vi "LV2017CP.vi"() -> ()   [LabVIEW 2016]
doc: "This example performs a serial port write and a serial port read. The parameters set for the serial port must match the parameters of the connected instrument or device. The VISA Configure Serial Port VI sets the configuration parameters. The front panel displays the controls used to configure the basic parameters, such as baud rate, data bits, and parity. The VI passes the VISA resource name to other VIs that perform operations on that VISA resource. The VISA Write function sends a command to the serial device and the VISA Read function returns data based on the command. The VISA Close function then closes the reference to the serial device. It is important to close the reference; otherwise, further communication through that port might not be possible."
uses:
  <vilib>/Instr/_visa.llb/VISA Configure Serial Port (Instr).vi
  Serial - Settings.ctl
panel:
  in  "Tyre Diameter(m) 2":sgl=0.5
  in  "Name your log file:":string="09_12_2019"
  in  "Error Cancellation (Def:On)":bool
  out "Answer to Write Command 2":string
  out "Speed Reference":sgl(graph)=57.306286
  out "Speed Ref in 21202":string
  out "Floating Point 5":sgl
  out "Speed Ref in 21201":string
  in  "write buffer 5":string="\u0002\u0003RÑ\u0000\u0002„¹"
  out "Floating Point 4":sgl
  out "Speed Ref in 21201":string
  in  "write buffer 4":string="\u0002\u0003RÐ\u0000\u0002Õy"
  in  "write buffer 3":string="\u0002\u0003I<\u0000\u0002\u0012h"
  out "read buffer 6":string
  out "read buffer 5":string
  out "read buffer 4":string
  out "read buffer 3":string
  out "read buffer 2":string
  out "read buffer":string
  in  "write buffer 2":string="\u0002\u0003RÏ\u0000\u0002ä¿"
  in  "write buffer":string="\u0002\u0010RÏ\u0000\u0002\u0004\u0000\u0000@ d "
  out "Answer to Write Command":string
  out "Floating Point 3":sgl=5.00679
  out "Speed Ref in 21200":string
  out "Floating Point 2":sgl=0.14305113
  out "Speed Ref in Monitor":string
  out "I_d":sgl(graph)=0.08283757
  out "I_q":sgl(graph)=-0.08283757
  out "Power(kW)":sgl(graph)=8.934696e-07
  out "Current(I)":sgl(graph)
  in  "file path (dialog if empty)":path=path "C:/Users/arda/Desktop/Thesis/random.txt"
  in  "Tyre Diameter(m)":sgl=0.5
  out "Measured RPM":sgl(graph)
  in  "Enum":T1(ring)=enum."Default"
  in  "Continuous Connection(Def:ON)":bool=TRUE
  out "Estimated Torque":sgl(graph)=-0.29821524
  in  "Finish session(Def:Off/False)":bool
  in  "Connectivity Check (Def:Off)":bool
  in  "timeout (10sec)":u32=10000
  out "connection check":u8[](array[numeric])=[0, 0, 0, 2]
  in  "Enable Termination\nChar (T)":bool
  in  "connection_verification":string="\u0002\u0003Fm\u0000\u0002@­"
  out "Serial Settings:Wire Mode":i8(ring)=-128 items=["Unknown"=-1, "RS485/Wire4"=0, "RS485/Wire2-EchoDTR"=1, "RS485/Wire2-CtrlDTR"=2, "RS485/Wire2-Auto"=3, "RS232/DTE"=-128, "RS232/DCE"=-127, "RS232/Auto"=-126]
  out "message":string="No Error"
  in  "Serial Settings":T2={"baud rate"=19200, "data bits"=8, "parity"=enum."Even", "stop bits"=10, "flow control"=0} {"flow control" items=["None"=0, "XON/XOFF"=1, "RTS/CTS"=2, "DTR/DSR"=4]; "stop bits" items=["1.0"=10, "1.5"=15, "2.0"=20]; "data bits" min=5 max=8 step=1; "baud rate" items=["75"=75, "110"=110, "134"=134, "150"=150, "300"=300, "600"=600, "1200"=1200, "1800"=1800, "2400"=2400, "4800"=4800, "9600"=7200, "19600"=9600, "14400"=14400, "19200"=19200, "28800"=28800, "38400"=38400, "56000"=56000, "57600"=57600, "115200"=115200, "128000"=128000, "230400"=230400]}
  in  "VISA resource name":refnum<visa-resource-name>="COM8"
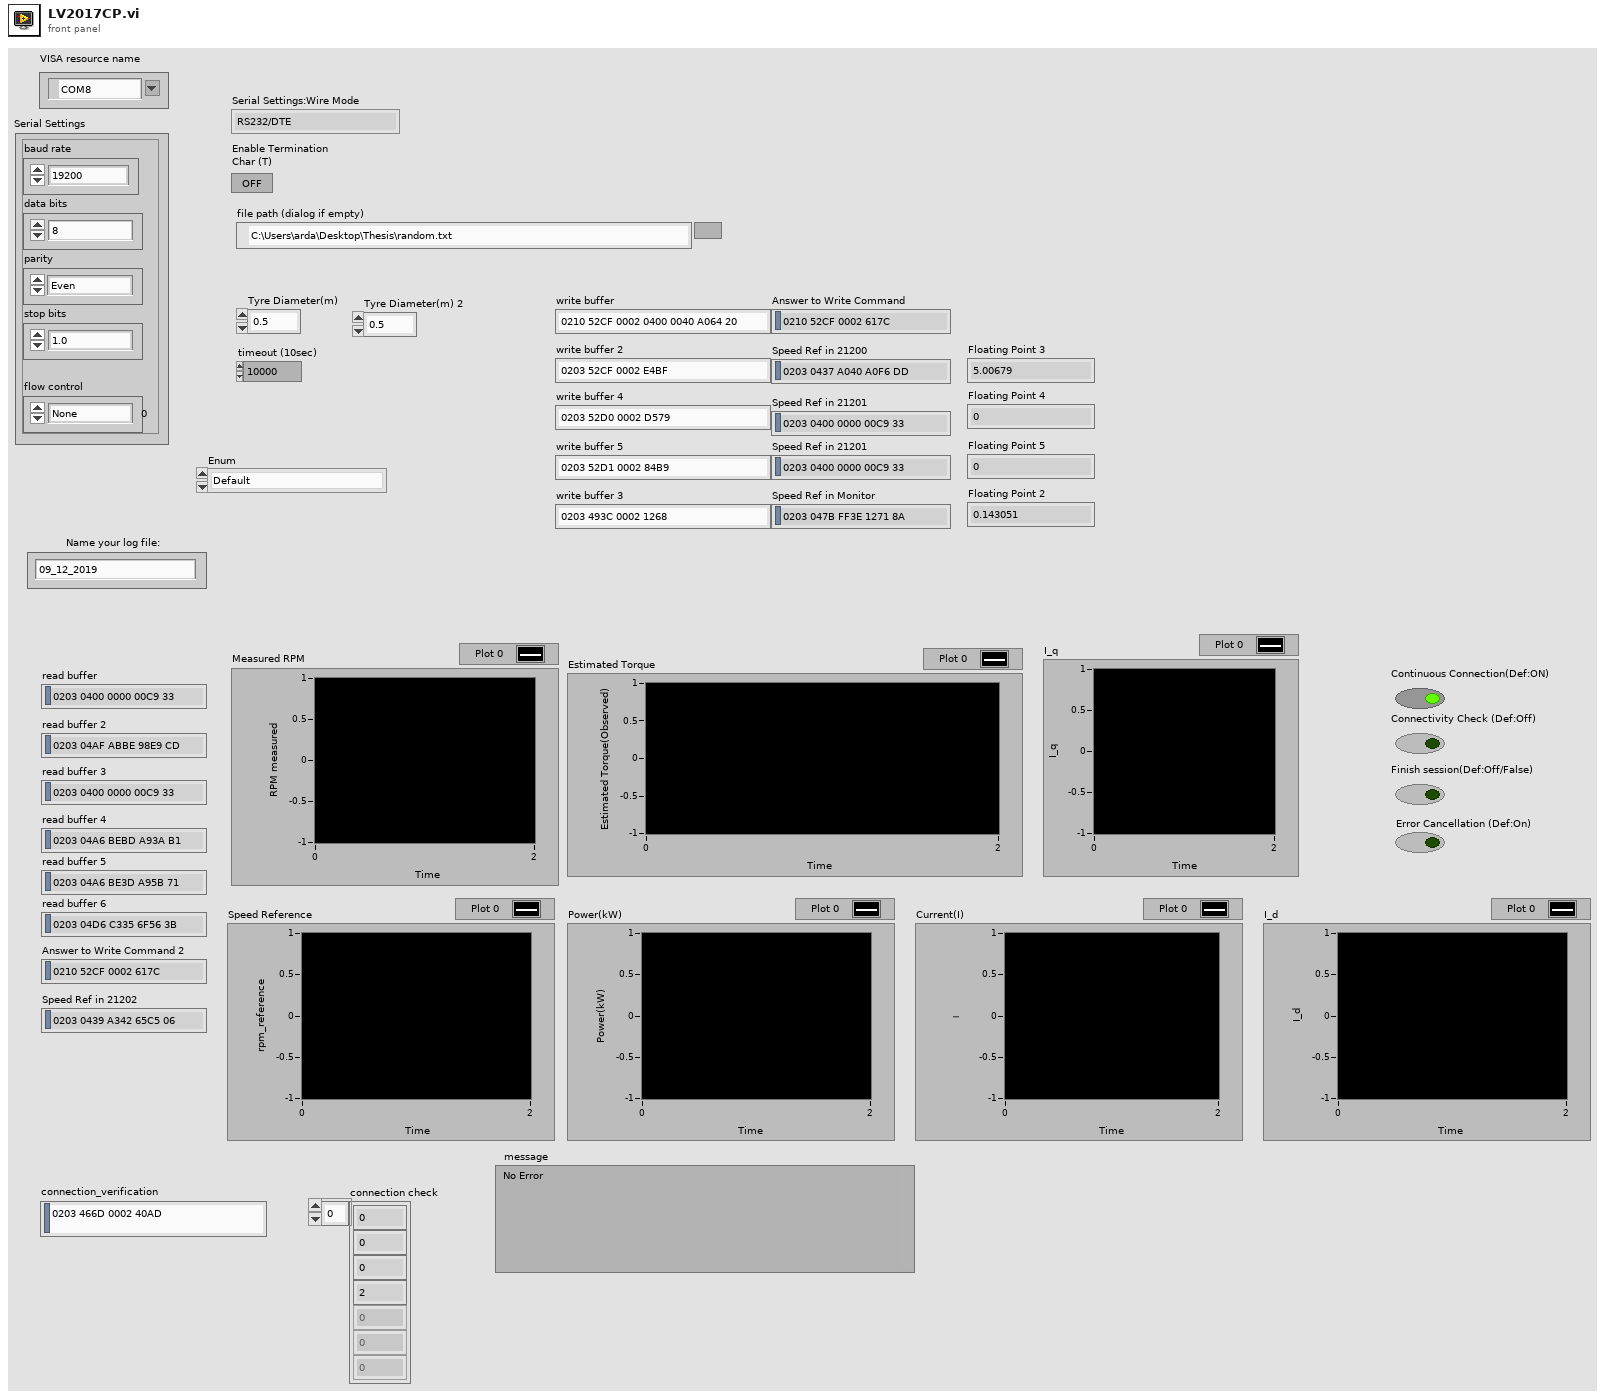
[diagram p1: front panel]
types:
  T1 = enum16{"Single Signal Trials", "Default", "Alarm Reset", "Write Save Command", "Drive Reset"}
  T2 = typedef "Serial - Settings.ctl" = cluster{"baud rate":u32, "data bits":u16, "parity":enum16{"None", "Odd", "Even", "Mark", "Space"}, "stop bits":u16, "flow control":u16}
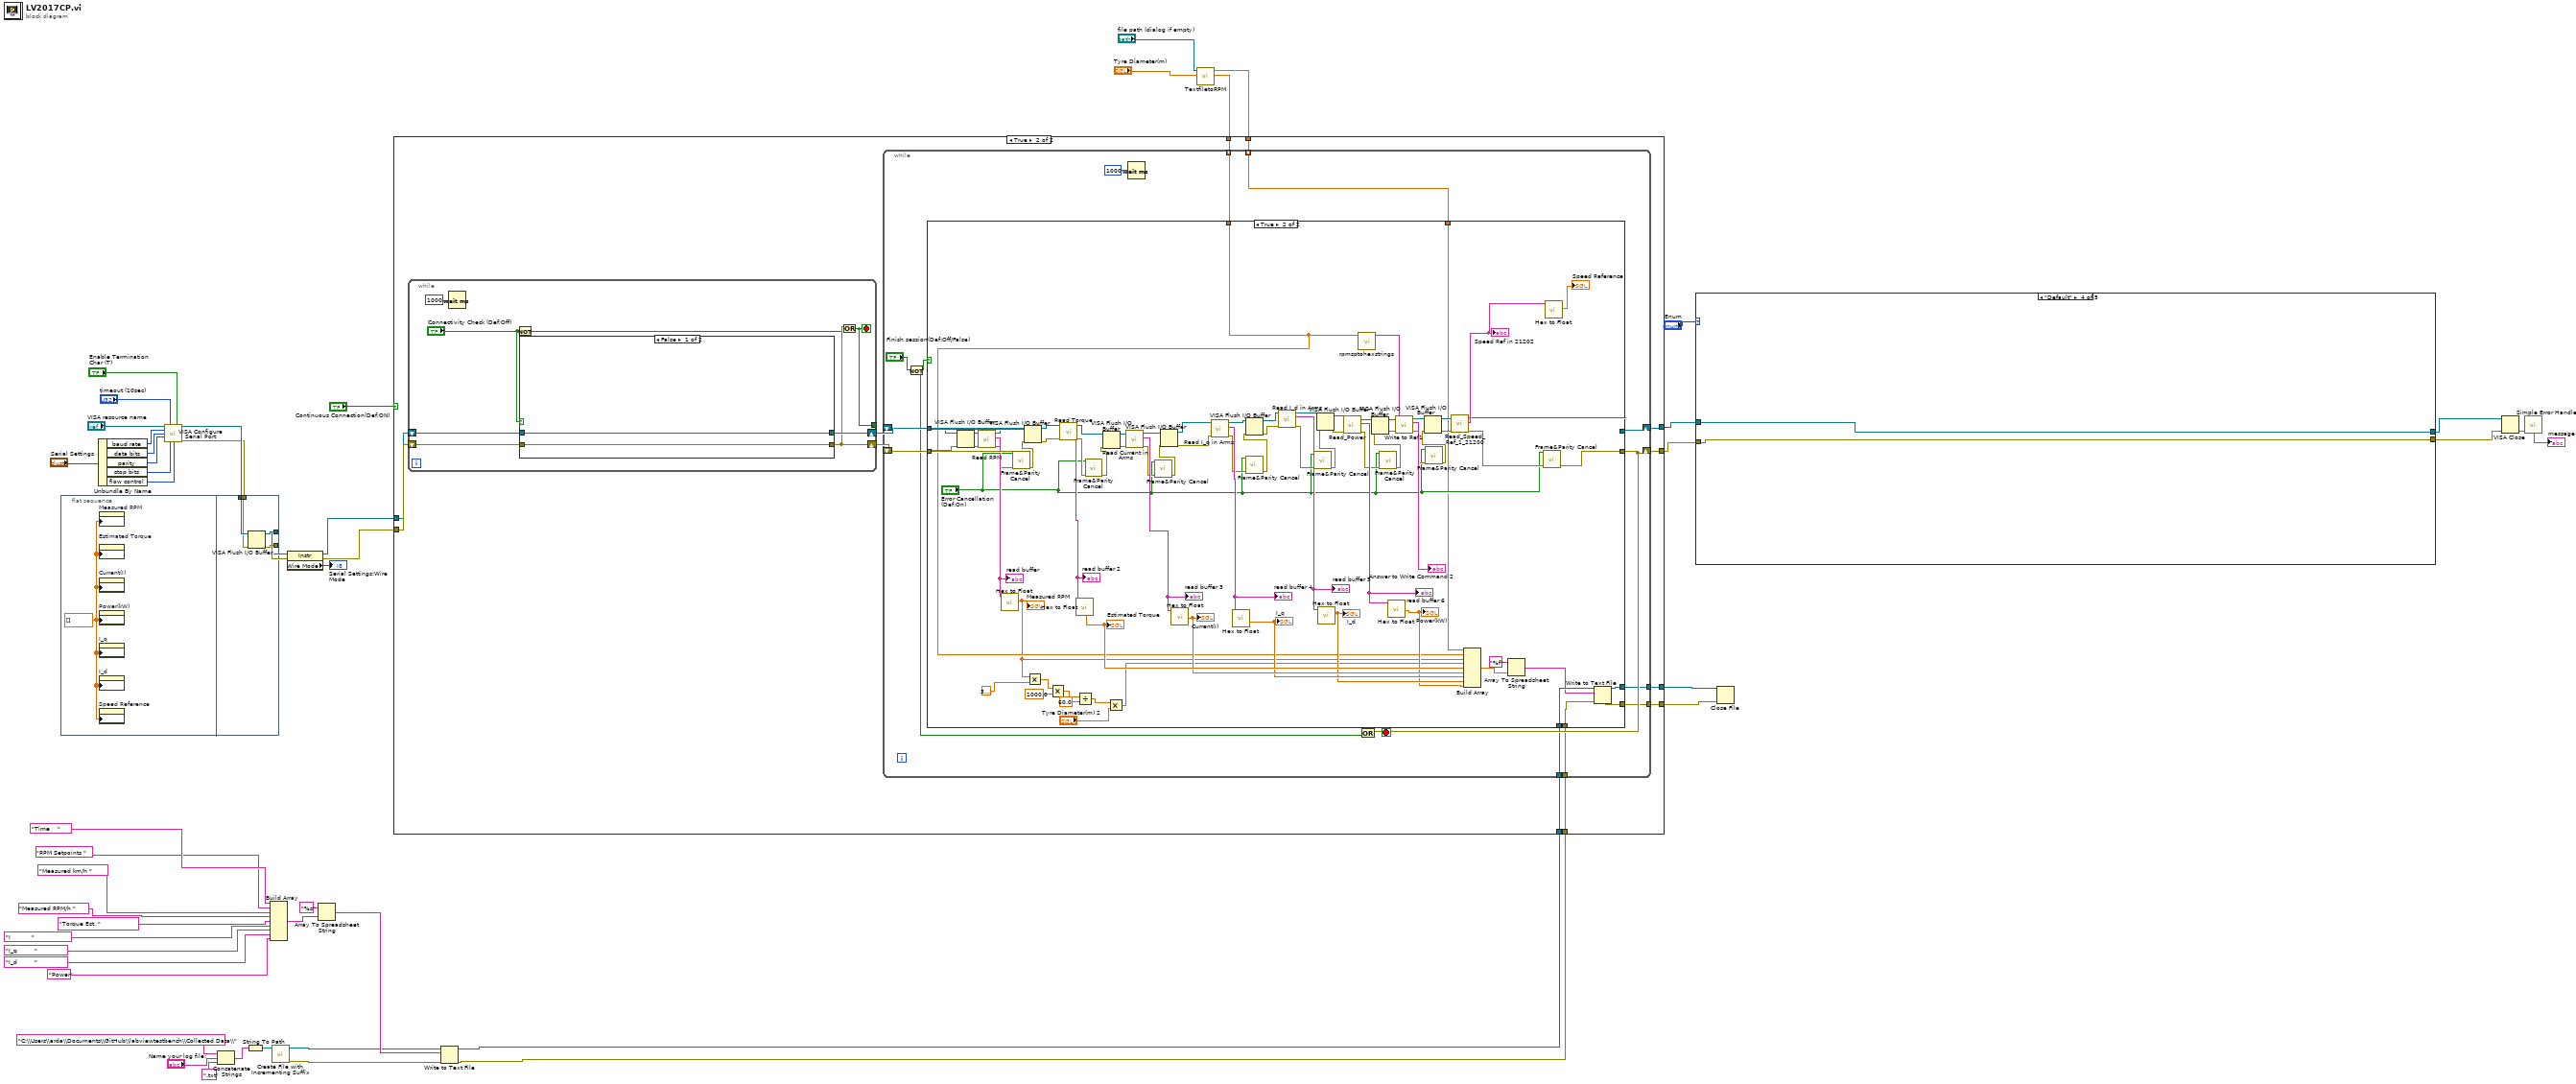
[diagram p0: block diagram]
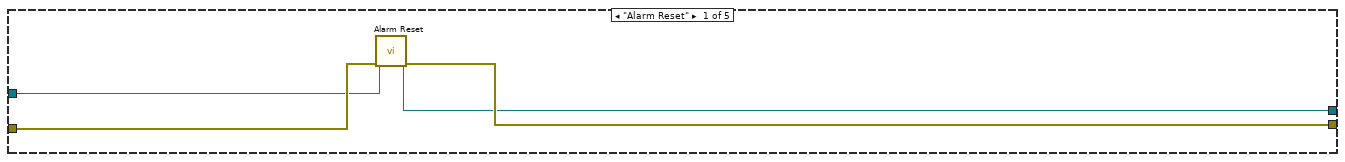
[diagram p2: hidden frame]
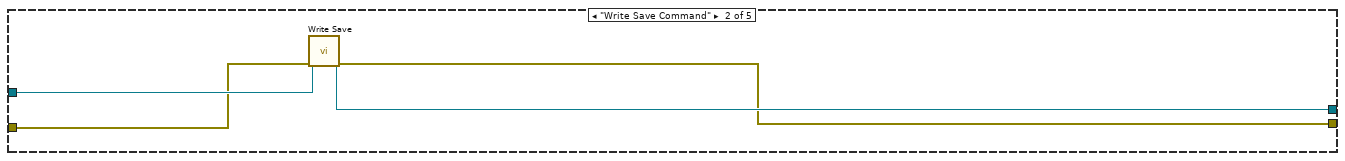
[diagram p3: hidden frame]
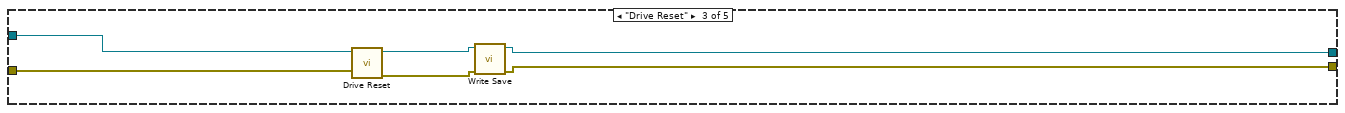
[diagram p4: hidden frame]
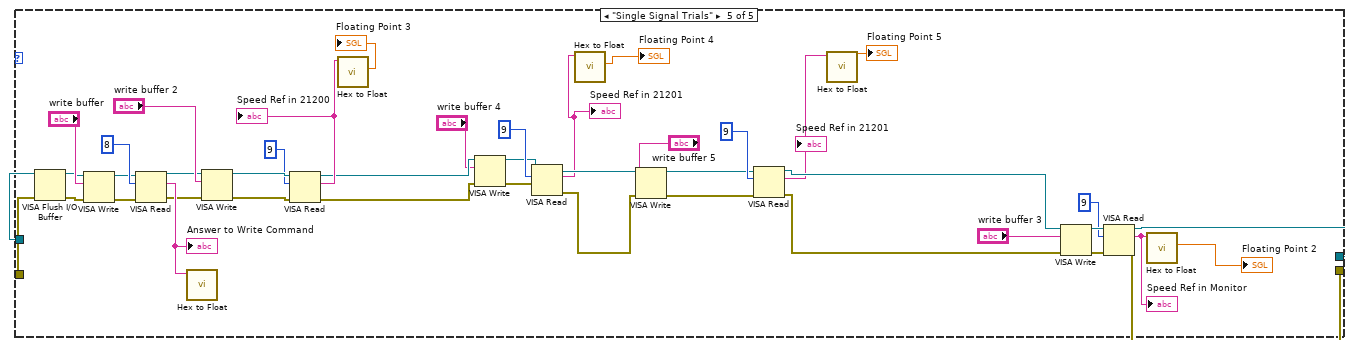
[diagram p5: hidden frame]
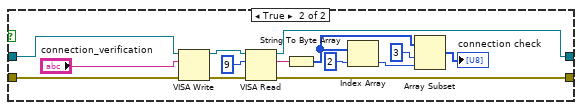
[diagram p7: hidden frame]
diagram:
  n1 = flat-sequence {
    tunnel: [w56] -> w42
    tunnel: [w55] -> w41
    tunnel: w40 -> [w54]
    tunnel: w39 -> [w53]
    frame #0 {
      w52 = sgl[] [] ("History Data")
      n2 = property on="Measured RPM" class="WFChart (strict)"("History Data"=w52) -> ()  [unwired: 2 in, 2 out]
      n3 = property on="Estimated Torque" class="WFChart (strict)"("History Data"=w52) -> ()  [unwired: 2 in, 2 out]
      n4 = property on="Current(I)" class="WFChart (strict)"("History Data"=w52) -> ()  [unwired: 2 in, 2 out]
      n5 = property on="Power(kW)" class="WFChart (strict)"("History Data"=w52) -> ()  [unwired: 2 in, 2 out]
      n6 = property on="I_q" class="WFChart (strict)"("History Data"=w52) -> ()  [unwired: 2 in, 2 out]
      n7 = property on="I_d" class="WFChart (strict)"("History Data"=w52) -> ()  [unwired: 2 in, 2 out]
      n8 = property on="Speed Reference" class="WFChart (strict)"("History Data"=w52) -> ()  [unwired: 2 in, 2 out]
    }
    frame #1 {
      n9 = VISA Flush I/O Buffer(VISA resource name=w54, error in (no error)=w53) -> (VISA resource name out=w55:refnum<visa-resource-name>, error out=w56:errorcluster)  [unwired: 1 in]
    }
  }
  n10 = Unbundle By Name("Serial Settings") -> ("baud rate"=w45:u32, "data bits"=w49:u16, "parity"=w48:enum16{"None", "Odd", "Even", "Mark", "Space"}, "stop bits"=w47:u16, "flow control"=w46:u16)
  n11 = call-poly "VISA Configure Serial Port"("VISA resource name"="VISA resource name", "timeout (10sec)"="timeout (10sec)", "Enable Termination\nChar (T)"="Enable Termination\nChar (T)", "baud rate (9600)"=w45, "data bits (8)"=w49, "parity (0:none)"=w48, "stop bits (10: 1 bit)"=w47, "flow control (0:none)"=w46) -> ("VISA resource name out"=w40:refnum<visa-resource-name>, "error out"=w39:errorcluster)  [unwired: 1 in, 5 out]
  n12 = Concatenate Strings("C:\\Users\\arda\\Documents\\GitHub\\labviewtestbench\\Collected Data\\" ("string"), "Name your log file:", ".txt") -> (w19:string)
  n13 = String To Path(string=w19) -> (path=w15:path)
  n14 = Build Array("Time    " ("element"), "RPM Setpoints ", "Measured km/h ", "Measured RPM/h ", "Torque Est. ", "I           " ("element"), "I_q         " ("element"), "I_d         " ("element"), "Power" ("element")) -> (w22:string[])
  n15 = call <vilib>:"Create File with Incrementing Suffix.vi"("file path"=w15) -> ("error out"=w13:errorcluster, "refnum out"=w14:refnum<file>)  [unwired: 8 in, 1 out]
  n16 = property class="Instr"(reference=w41, error in=w42) -> (reference out=w36:refnum<visa-resource-name>, error out=w37:errorcluster, "Wire Mode"=→"Serial Settings:Wire Mode":i16)
  n17 = Array To Spreadsheet String(array=w22, 3:"%s" ("format string")) -> (spreadsheet string=w20:string)  [unwired: 1 in]
  n18 = Write to Text File(file (use dialog)=w14, text=w20, error in=w13) -> (refnum out=w6:refnum<file>, error out=w7:errorcluster)  [unwired: 1 in, 1 out]
  n19 = call "TextfiletoRPM.vi"("Tyre Diameter(m)"="Tyre Diameter(m)", "file path (dialog if empty)"="file path (dialog if empty)") -> ("Array"=w28:dbl[], "time_sp"=w5:sgl[])  [unwired: 8 in]
  n20 = case shown="True" "Continuous Connection(Def:ON)" {
    tunnel: w37 -> [w59 w72]
    tunnel: w36 -> [w60 w71]
    tunnel: [w60 w68] -> w33
    tunnel: w28 -> [_ w67]
    tunnel: [w59 w66] -> w25
    tunnel: w6 -> [w57 w65]
    tunnel: w7 -> [w58 w64]
    tunnel: [w57 w63] -> w24
    tunnel: [w58 w62] -> w23
    tunnel: w5 -> [_ w61]
    frame False {
    }
    frame True {
      n21 = while {
        shift-right: [w80] -> w70
        shift-left: w71 -> [w79]
        shift-right: [w77] -> w69
        shift-left: w72 -> [w78]
        tunnel: [w73] -> _
        stop <- w73 stop-if-true
        n22 = Wait (ms)(milliseconds to wait=u32 1000) -> ()  [unwired: 1 out]
        n23 = Not(x="Connectivity Check (Def:Off)") -> (.not. x?=w74:bool)
        n24 = case shown="False" "Connectivity Check (Def:Off)" {
          tunnel: [w82 w96] -> w80
          tunnel: w79 -> [w82 w95]
          tunnel: w78 -> [w81 w94]
          tunnel: [w81 w93] -> w77
          frame False {
          }
          frame True {
            n25 = VISA Write(VISA resource name=w95, write buffer="connection_verification", error in (no error)=w94) -> (VISA resource name out=w92:refnum<visa-resource-name>, error out=w90:errorcluster)  [unwired: 1 out]
            n26 = VISA Read(VISA resource name=w92, byte count=u32 9, error in (no error)=w90) -> (VISA resource name out=w96:refnum<visa-resource-name>, read buffer=w84:string, error out=w93:errorcluster)  [unwired: 1 out]
            n27 = String To Byte Array(string=w84) -> (unsigned byte array=w88:u8[])
            n28 = Index Array(array=w88, index=2) -> (element=w85:u8)
            n29 = Array Subset(array=w88, index=3 ("length"), length=w85) -> (→"connection check":u8[])
          }
        }
        n30 = Or(x=w77, y=w74) -> (x .or. y?=w73:bool)
      }
      n31 = while {
        shift-right: [w108] -> w68
        shift-left: w70 -> [w110]
        shift-right: [w106] -> w66
        shift-left: w69 -> [w109]
        tunnel: w67 -> [w104] mode=indexing
        tunnel: w65 -> [w101]
        tunnel: w64 -> [w100]
        tunnel: [w99] -> w63
        tunnel: [w98] -> w62
        tunnel: w61 -> [w97] mode=indexing
        stop <- w105 stop-if-true
        n32 = Not(x="Finish session(Def:Off/False)") -> (.not. x?=w103:bool)
        n33 = case shown="True" w103 {
          tunnel: w110 -> [w114 w183]
          tunnel: w109 -> [w113 w181]
          tunnel: [w114 w177] -> w108
          tunnel: [w113 w184] -> w106
          tunnel: w104 -> [_ w117]
          tunnel: w101 -> [w112 w130]
          tunnel: w100 -> [w111 w129]
          tunnel: [w112 w128] -> w99
          tunnel: [w111 w127] -> w98
          tunnel: w97 -> [_ w118]
          frame False {
          }
          frame True {
            n34 = VISA Flush I/O Buffer(VISA resource name=w183, error in (no error)=w181) -> (VISA resource name out=w182:refnum<visa-resource-name>, error out=w174:errorcluster)  [unwired: 1 in]
            n35 = call "Read RPM.vi"("error in (no error)"=w174, "VISA resource name"=w182) -> ("error out"=w152:errorcluster, "read buffer"=w189:string, "VISA resource name out"=w173:refnum<visa-resource-name>)  [unwired: 7 in]
            "read buffer" <- w189
            n36 = call "Hex to Float.vi"("read buffer in"=w189) -> ("Floating Point"=w116:sgl)  [unwired: 9 in, 1 out]
            "Measured RPM" <- w116
            n37 = call "Frame&Parity Cancel.vi"("error in (no error)"=w152, "Error Cancellation (Def:On)"="Error Cancellation (Def:On)") -> ("error out"=w151:errorcluster)  [unwired: 9 in]
            n38 = VISA Flush I/O Buffer(VISA resource name=w173, error in (no error)=w151) -> (VISA resource name out=w172:refnum<visa-resource-name>, error out=w171:errorcluster)  [unwired: 1 in]
            n39 = Multiply(x=w116, y=3.141592653589793) -> (x*y=w124:dbl)
            n40 = Multiply(x=w124, y=1000.0) -> (x*y=w122:dbl)
            n41 = call "Read Torque.vi"("error in (no error)"=w171, "VISA Refnum in"=w172) -> ("error out"=w150:errorcluster, "read buffer"=w190:string, "VISA Refnum out"=w170:refnum<visa-resource-name>)  [unwired: 7 in]
            "read buffer 2" <- w190
            n42 = call "Hex to Float.vi"("read buffer in"=w190) -> ("Floating Point"=w137:sgl)  [unwired: 9 in, 1 out]
            "Estimated Torque" <- w137
            n43 = Divide(x=w122, y=60.0) -> (x/y=w120:dbl)
            n44 = call "Frame&Parity Cancel.vi"("error in (no error)"=w150, "Error Cancellation (Def:On)"="Error Cancellation (Def:On)") -> ("error out"=w149:errorcluster)  [unwired: 9 in]
            n45 = VISA Flush I/O Buffer(VISA resource name=w170, error in (no error)=w149) -> (VISA resource name out=w168:refnum<visa-resource-name>, error out=w169:errorcluster)  [unwired: 1 in]
            n46 = Multiply(x=w120, y="Tyre Diameter(m) 2") -> (x*y=w115:dbl)
            n47 = call "Read Current in Arms.vi"("error in (no error)"=w169, "VISA Refnum in"=w168) -> ("error out"=w148:errorcluster, "read buffer"=w187:string, "VISA Refnum out"=w167:refnum<visa-resource-name>)  [unwired: 7 in]
            "read buffer 3" <- w187
            n48 = call "Frame&Parity Cancel.vi"("error in (no error)"=w148, "Error Cancellation (Def:On)"="Error Cancellation (Def:On)") -> ("error out"=w147:errorcluster)  [unwired: 9 in]
            n49 = VISA Flush I/O Buffer(VISA resource name=w167, error in (no error)=w147) -> (VISA resource name out=w166:refnum<visa-resource-name>, error out=w165:errorcluster)  [unwired: 1 in]
            n50 = call "Hex to Float.vi"("read buffer in"=w187) -> ("Floating Point"=w136:sgl)  [unwired: 9 in, 1 out]
            "Current(I)" <- w136
            n51 = call "Read I_q in Arms.vi"("error in (no error)"=w165, "VISA Refnum in"=w166) -> ("error out"=w146:errorcluster, "read buffer"=w186:string, "VISA Refnum out"=w162:refnum<visa-resource-name>)  [unwired: 7 in]
            "read buffer 4" <- w186
            n52 = call "Hex to Float.vi"("read buffer in"=w186) -> ("Floating Point"=w135:sgl)  [unwired: 9 in, 1 out]
            "I_q" <- w135
            n53 = call "Frame&Parity Cancel.vi"("error in (no error)"=w146, "Error Cancellation (Def:On)"="Error Cancellation (Def:On)") -> ("error out"=w145:errorcluster)  [unwired: 9 in]
            n54 = VISA Flush I/O Buffer(VISA resource name=w162, error in (no error)=w145) -> (VISA resource name out=w163:refnum<visa-resource-name>, error out=w164:errorcluster)  [unwired: 1 in]
            n55 = call "Read I_d in Arms.vi"("error in (no error)"=w164, "VISA Refnum in"=w163) -> ("error out"=w144:errorcluster, "read buffer"=w185:string, "VISA Refnum out"=w161:refnum<visa-resource-name>)  [unwired: 7 in]
            "read buffer 5" <- w185
            n56 = call "Frame&Parity Cancel.vi"("error in (no error)"=w144, "Error Cancellation (Def:On)"="Error Cancellation (Def:On)") -> ("error out"=w143:errorcluster)  [unwired: 9 in]
            n57 = VISA Flush I/O Buffer(VISA resource name=w161, error in (no error)=w143) -> (VISA resource name out=w159:refnum<visa-resource-name>, error out=w160:errorcluster)  [unwired: 1 in]
            n58 = call "Hex to Float.vi"("read buffer in"=w185) -> ("Floating Point"=w134:sgl)  [unwired: 9 in, 1 out]
            "I_d" <- w134
            n59 = call "Read_Power.vi"("error in (no error)"=w160, "VISA Refnum in"=w159) -> ("error out"=w142:errorcluster, "read buffer"=w188:string, "VISA Refnum out"=w158:refnum<visa-resource-name>)  [unwired: 7 in]
            "read buffer 6" <- w188
            n60 = call "rpmsptohexstrings.vi"("RPM value"=w117) -> ("String out"=w175:string)  [unwired: 10 in]
            n61 = call "Frame&Parity Cancel.vi"("error in (no error)"=w142, "Error Cancellation (Def:On)"="Error Cancellation (Def:On)") -> ("error out"=w141:errorcluster)  [unwired: 9 in]
            n62 = VISA Flush I/O Buffer(VISA resource name=w158, error in (no error)=w141) -> (VISA resource name out=w157:refnum<visa-resource-name>, error out=w156:errorcluster)  [unwired: 1 in]
            n63 = call "Hex to Float.vi"("read buffer in"=w188) -> ("Floating Point"=w133:sgl)  [unwired: 9 in, 1 out]
            "Power(kW)" <- w133
            n64 = call "Write to Ref1.vi"("error in (no error)"=w156, "String in"=w175, "VISA Refnum in"=w157) -> ("error out"=w140:errorcluster, "read buffer"=→"Answer to Write Command 2":string, "VISA Refnum out"=w155:refnum<visa-resource-name>)  [unwired: 6 in]
            n65 = call "Frame&Parity Cancel.vi"("error in (no error)"=w140, "Error Cancellation (Def:On)"="Error Cancellation (Def:On)") -> ("error out"=w139:errorcluster)  [unwired: 9 in]
            n66 = VISA Flush I/O Buffer(VISA resource name=w155, error in (no error)=w139) -> (VISA resource name out=w154:refnum<visa-resource-name>, error out=w153:errorcluster)  [unwired: 1 in]
            n67 = call "Read_Speed_Ref_1_21200.vi"("error in (no error)"=w153, "VISA Refnum in"=w154) -> ("error out"=w176:errorcluster, "read buffer"=w180:string, "VISA Refnum out"=w177:refnum<visa-resource-name>)  [unwired: 7 in]
            "Speed Ref in 21202" <- w180
            n68 = Build Array(w118, w117, w116, w115, w137, w136, w135, w134, w133) -> (w132:dbl[])
            n69 = Array To Spreadsheet String(array=w132, 3:"%f" ("format string")) -> (spreadsheet string=w126:string)  [unwired: 1 in]
            n70 = call "Frame&Parity Cancel.vi"("error in (no error)"=w176, "Error Cancellation (Def:On)"="Error Cancellation (Def:On)") -> ("error out"=w184:errorcluster)  [unwired: 9 in]
            n71 = call "Hex to Float.vi"("read buffer in"=w180) -> ("Floating Point"=→"Speed Reference":sgl)  [unwired: 9 in, 1 out]
            n72 = Write to Text File(file (use dialog)=w130, text=w126, error in=w129) -> (refnum out=w128:refnum<file>, error out=w127:errorcluster)  [unwired: 1 in, 1 out]
          }
        }
        n73 = Wait (ms)(milliseconds to wait=u32 1000) -> ()  [unwired: 1 out]
        n74 = Or(x=w106, y="Finish session(Def:Off/False)") -> (x .or. y?=w105:bool)
      }
    }
  }
  n75 = case shown="\"Default\"" "Enum" {
    tunnel: w25 -> [w194 w197 w203 w205 w246]
    tunnel: w33 -> [w193 w198 w204 w206 w247]
    tunnel: [w192 w195 w199 w205 w248] -> w32
    tunnel: [w191 w196 w200 w206 w249] -> w31
    frame "Alarm Reset" {
      n76 = call "Alarm Reset.vi"("error in (no error)"=w194, "VISA Refnum in"=w193) -> ("error out"=w192:errorcluster, "VISA Refnum out"=w191:refnum<visa-resource-name>)  [unwired: 7 in, 1 out]
    }
    frame "Write Save Command" {
      n77 = call "Write Save.vi"("error in (no error)"=w197, "VISA Refnum in"=w198) -> ("error out"=w195:errorcluster, "VISA Refnum out"=w196:refnum<visa-resource-name>)  [unwired: 7 in, 1 out]
    }
    frame "Drive Reset" {
      n78 = call "Drive Reset.vi"("error in (no error)"=w203, "VISA Refnum in"=w204) -> ("error out"=w201:errorcluster, "VISA Refnum out"=w202:refnum<visa-resource-name>)  [unwired: 7 in, 1 out]
      n79 = call "Write Save.vi"("error in (no error)"=w201, "VISA Refnum in"=w202) -> ("error out"=w199:errorcluster, "VISA Refnum out"=w200:refnum<visa-resource-name>)  [unwired: 7 in, 1 out]
    }
    frame "Default" {
    }
    frame "Single Signal Trials" {
      n80 = VISA Flush I/O Buffer(VISA resource name=w247, error in (no error)=w246) -> (VISA resource name out=w228:refnum<visa-resource-name>, error out=w229:errorcluster)  [unwired: 1 in]
      n81 = VISA Write(VISA resource name=w228, write buffer="write buffer", error in (no error)=w229) -> (VISA resource name out=w231:refnum<visa-resource-name>, error out=w230:errorcluster)  [unwired: 1 out]
      n82 = VISA Read(VISA resource name=w231, byte count=u32 8, error in (no error)=w230) -> (VISA resource name out=w227:refnum<visa-resource-name>, read buffer=w232:string, error out=w226:errorcluster)  [unwired: 1 out]
      "Answer to Write Command" <- w232
      n83 = call "Hex to Float.vi"("read buffer in"=w232) -> ()  [unwired: 9 in, 2 out]
      n84 = VISA Write(VISA resource name=w227, write buffer="write buffer 2", error in (no error)=w226) -> (VISA resource name out=w237:refnum<visa-resource-name>, error out=w238:errorcluster)  [unwired: 1 out]
      n85 = VISA Read(VISA resource name=w237, byte count=u32 9, error in (no error)=w238) -> (VISA resource name out=w223:refnum<visa-resource-name>, read buffer=w235:string, error out=w222:errorcluster)  [unwired: 1 out]
      "Speed Ref in 21200" <- w235
      n86 = call "Hex to Float.vi"("read buffer in"=w235) -> ("Floating Point"=→"Floating Point 3":sgl)  [unwired: 9 in, 1 out]
      n87 = VISA Write(VISA resource name=w223, write buffer="write buffer 4", error in (no error)=w222) -> (VISA resource name out=w221:refnum<visa-resource-name>, error out=w220:errorcluster)  [unwired: 1 out]
      n88 = VISA Read(VISA resource name=w221, byte count=u32 9, error in (no error)=w220) -> (VISA resource name out=w215:refnum<visa-resource-name>, read buffer=w211:string, error out=w216:errorcluster)  [unwired: 1 out]
      "Speed Ref in 21201" <- w211
      n89 = call "Hex to Float.vi"("read buffer in"=w211) -> ("Floating Point"=→"Floating Point 4":sgl)  [unwired: 9 in, 1 out]
      n90 = VISA Write(VISA resource name=w215, write buffer="write buffer 5", error in (no error)=w216) -> (VISA resource name out=w218:refnum<visa-resource-name>, error out=w217:errorcluster)  [unwired: 1 out]
      n91 = VISA Read(VISA resource name=w218, byte count=u32 9, error in (no error)=w217) -> (VISA resource name out=w213:refnum<visa-resource-name>, read buffer=w207:string, error out=w214:errorcluster)  [unwired: 1 out]
      "Speed Ref in 21201" <- w207
      n92 = call "Hex to Float.vi"("read buffer in"=w207) -> ("Floating Point"=→"Floating Point 5":sgl)  [unwired: 9 in, 1 out]
      n93 = VISA Write(VISA resource name=w213, write buffer="write buffer 3", error in (no error)=w214) -> (VISA resource name out=w243:refnum<visa-resource-name>, error out=w244:errorcluster)  [unwired: 1 out]
      n94 = VISA Read(VISA resource name=w243, byte count=u32 9, error in (no error)=w244) -> (VISA resource name out=w249:refnum<visa-resource-name>, read buffer=w242:string, error out=w248:errorcluster)  [unwired: 1 out]
      "Speed Ref in Monitor" <- w242
      n95 = call "Hex to Float.vi"("read buffer in"=w242) -> ("Floating Point"=→"Floating Point 2":sgl)  [unwired: 9 in, 1 out]
    }
  }
  n96 = Close File(refnum=w24, error in=w23) -> ()  [unwired: 2 out]
  n97 = VISA Close(VISA resource name=w31, error in (no error)=w32) -> (error out=w35:errorcluster)
  n98 = call <vilib>:"Simple Error Handler.vi"("error in (no error)"=w35) -> ("message"=→"message":string)  [unwired: 1 in, 7 out]
